vi "xhochy.vi"(8 "Base":dbl format="%#_13g", 11 "Exponent":i32) -> (0 "result":dbl)   [LabVIEW 2013, in "Utilities.lvlib"]
uses:
  Utilities.lvlib
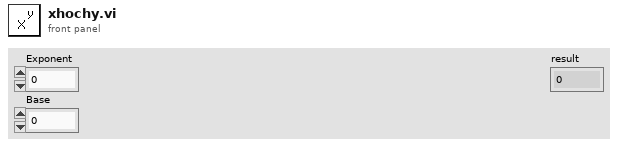
[diagram p1: front panel]
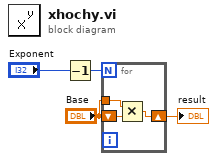
[diagram p0: block diagram]
diagram:
  n1 = Decrement(x="Exponent") -> (x-1=w1:i32)
  n2 = for {
    N: w1 -> [_]
    shift-right: [w7] -> w3
    shift-left: "Base" -> [w6]
    tunnel: "Base" -> [w5]
    n3 = Multiply(x=w5, y=w6) -> (x*y=w7:dbl)
  }
  "result" <- w3
